vi "day 11 task 1.vi"() -> ()   [LabVIEW 2019]
uses:
  <userlib>/_OpenG.lib/array/array.llb/Search 1D Array (I32)__ogtk.vi
panel:
  out "level of monkey business":i32
  out "Amount of inspections by each monkey":i32[](array[numeric])
  out "Monkeys after 20 rounds":T1(array[cluster])
  out "Monkeys":T2(array[cluster])
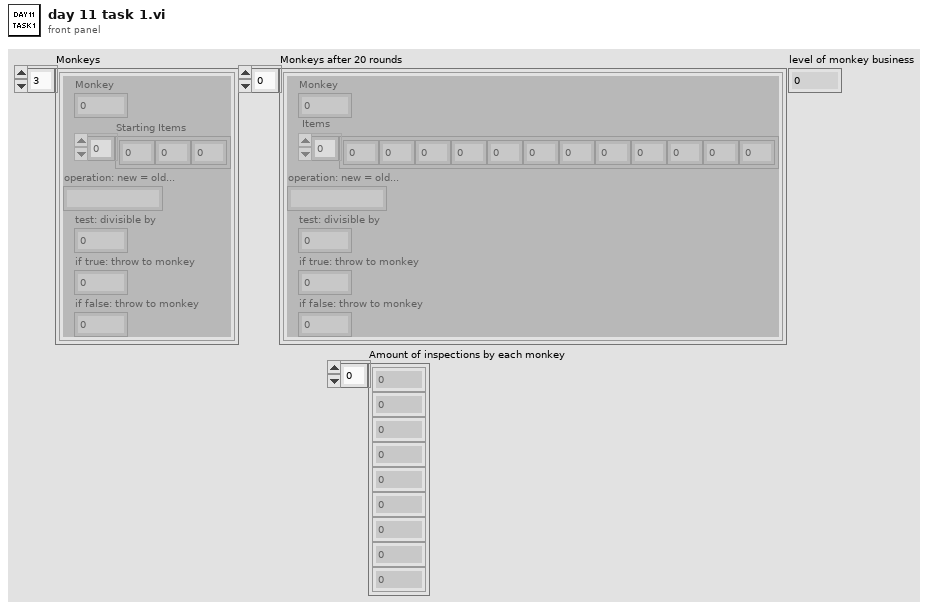
[diagram p1: front panel]
types:
  T1 = cluster{"Monkey":i32, " Items":i32[], "operation: new = old...":string, "test: divisible by":i32, "if true: throw to monkey":i32, "if false: throw to monkey":i32}[]
  T2 = cluster{"Monkey":i32, "Starting Items":i32[], "operation: new = old...":string, "test: divisible by":i32, "if true: throw to monkey":i32, "if false: throw to monkey":i32}[]
  T3 = cluster{"Monkey":i32, "Starting Items":i32[], "operation: new = old...":string, "test: divisible by":i32, "if true: throw to monkey":i32, "if false: throw to monkey":i32}
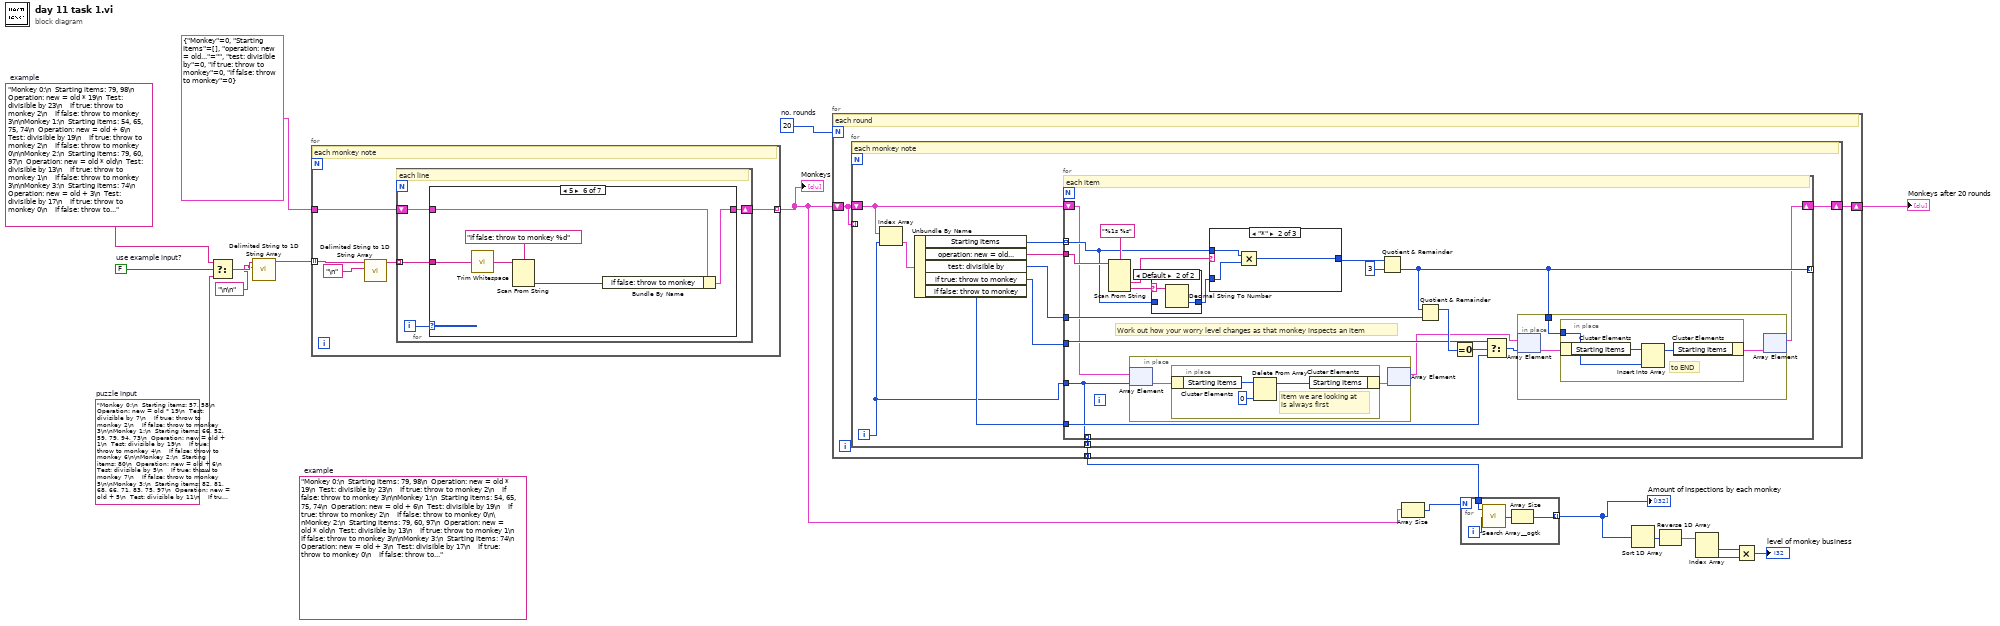
[diagram p0: block diagram]
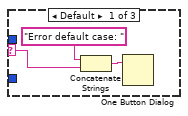
[diagram p3: hidden frame]
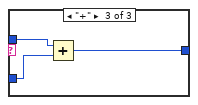
[diagram p4: hidden frame]
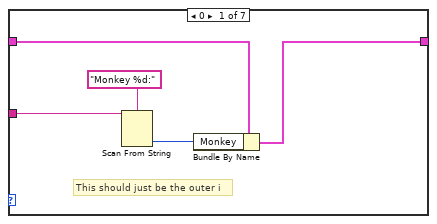
[diagram p5: hidden frame]
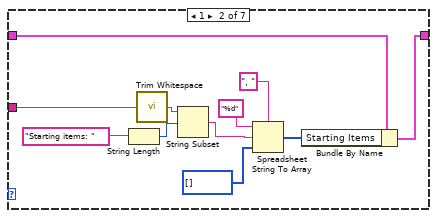
[diagram p6: hidden frame]
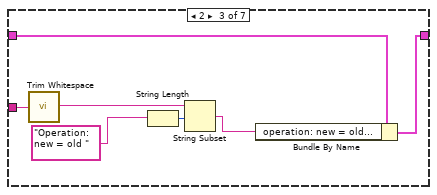
[diagram p7: hidden frame]
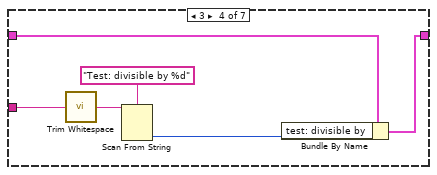
[diagram p8: hidden frame]
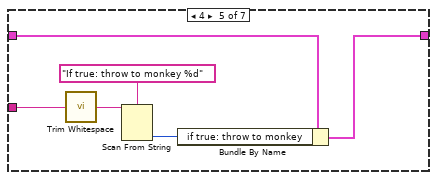
[diagram p9: hidden frame]
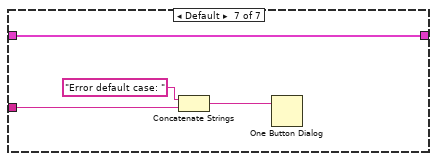
[diagram p10: hidden frame]
diagram:
  w10 = 20  # no. rounds
  (unwired) "Monkey 0:\n  Starting items: 79, 98\n  Operation: new = old * 19\n  Test: divisible by 23\n    If true: throw to monkey 2\n    If false: throw to monkey 3\n\nMonkey 1:\n  Starting items: 54, 65, 75, 74\n  Operation: new = old + 6\n  Test: divisible by 19\n    If true: throw to monkey 2\n    If false: throw to monkey 0\n\nMonkey 2:\n  Starting items: 79, 60, 97\n  Operation: new = old * old\n  Test: divisible by 13\n    If true: throw to monkey 1\n    If false: throw to monkey 3\n\nMonkey 3:\n  Starting items: 74\n  Operation: new = old + 3\n  Test: divisible by 17\n    If true: throw to monkey 0\n    If false: throw to monkey 1"  # example
  w16 = "Monkey 0:\n  Starting items: 79, 98\n  Operation: new = old * 19\n  Test: divisible by 23\n    If true: throw to monkey 2\n    If false: throw to monkey 3\n\nMonkey 1:\n  Starting items: 54, 65, 75, 74\n  Operation: new = old + 6\n  Test: divisible by 19\n    If true: throw to monkey 2\n    If false: throw to monkey 0\n\nMonkey 2:\n  Starting items: 79, 60, 97\n  Operation: new = old * old\n  Test: divisible by 13\n    If true: throw to monkey 1\n    If false: throw to monkey 3\n\nMonkey 3:\n  Starting items: 74\n  Operation: new = old + 3\n  Test: divisible by 17\n    If true: throw to monkey 0\n    If false: throw to monkey 1"  # example
  w17 = FALSE  # use example input?
  w18 = "Monkey 0:\n  Starting items: 57, 58\n  Operation: new = old * 19\n  Test: divisible by 7\n    If true: throw to monkey 2\n    If false: throw to monkey 3\n\nMonkey 1:\n  Starting items: 66, 52, 59, 79, 94, 73\n  Operation: new = old + 1\n  Test: divisible by 19\n    If true: throw to monkey 4\n    If false: throw to monkey 6\n\nMonkey 2:\n  Starting items: 80\n  Operation: new = old + 6\n  Test: divisible by 5\n    If true: throw to monkey 7\n    If false: throw to monkey 5\n\nMonkey 3:\n  Starting items: 82, 81, 68, 66, 71, 83, 75, 97\n  Operation: new = old + 5\n  Test: divisible by 11\n    If true: throw to monkey 5\n    If false: throw to monkey 2\n\nMonkey 4:\n  Starting items: 55, 52, 67, 70, 69, 94, 90\n  Operation: new = old * old\n  Test: divisible by 17\n    If true: throw to monkey 0\n    If false: throw to monkey 3\n\nMonkey 5:\n  Starting items: 69, 85, 89, 91\n  Operation: new = old + 7\n  Test: divisible by 13\n    If true: throw to monkey 1\n    If false: throw to monkey 7\n\nMonkey 6:\n  Starting items: 75, 53, 73, 52, 75\n  Operation: new = old * 7\n  Test: divisible by 2\n    If true: throw to monkey 0\n    If false: throw to monkey 4\n\nMonkey 7:\n  Starting items: 94, 60, 79\n  Operation: new = old + 2\n  Test: divisible by 3\n    If true: throw to monkey 1\n    If false: throw to monkey 6"  # puzzle input
  n1 = Select(t=w16, s=w17, f=w18) -> (s? t:f=w15:string)
  n2 = call <vilib>:"Delimited String to 1D String Array.vi"("delimiter"="\n\n" ("regular expression"), "delimited string"=w15) -> ("string array"=w13:string[])  [unwired: 9 in]
  n3 = for {
    tunnel: w13 -> [w23] mode=indexing
    tunnel: T3 {"Monkey"=0, "Starting Items"=[], "operation: new = old..."="", "test: divisible by"=0, "if true: throw to monkey"=0, "if false: throw to monkey"=0} -> [w22]
    tunnel: [w21] -> w8 mode=indexing
    # "each monkey note"
    n4 = call <vilib>:"Delimited String to 1D String Array.vi"("delimiter"="\n", "delimited string"=w23) -> ("string array"=w20:string[])  [unwired: 9 in]
    n5 = for {
      tunnel: w20 -> [w26] mode=indexing
      shift-right: [w25] -> w21
      shift-left: w22 -> [w24]
      i -> [w27]
      # "each line"
      n6 = case shown="5" w27 {
        tunnel: w26 -> [w32 w40 w50 w54 w60 w66 w70]
        tunnel: [w30 w37 w48 w51 w57 w63 w69] -> w25
        tunnel: w24 -> [w29 w38 w49 w52 w58 w65 w69]
        frame 0 {
          # "This should just be the outer i"
          n7 = Scan From String(format string="Monkey %d:", input string=w32) -> (output 1=w28:i32)  [unwired: 3 in, 3 out]
          n8 = Bundle By Name(cluster=w29, "Monkey"=w28) -> (w30:T3)
        }
        frame 1 {
          n9 = String Length(string="Starting items: " ("format string")) -> (length=w34:i32)
          n10 = call <vilib>:"Trim Whitespace.vi"("string"=w40) -> ("trimmed string"=w33:string)  [unwired: 1 in]
          n11 = String Subset(string=w33, offset (0)=w34) -> (substring=w36:string)  [unwired: 1 in]
          n12 = Spreadsheet String To Array(delimiter (Tab)=", ", format string="%d", spreadsheet string=w36, array type (2D Dbl)=i32[] []) -> (array=w39:i32[])
          n13 = Bundle By Name(cluster=w38, "Starting Items"=w39) -> (w37:T3)
        }
        frame 2 {
          n14 = call <vilib>:"Trim Whitespace.vi"("string"=w50) -> ("trimmed string"=w46:string)  [unwired: 1 in]
          n15 = String Length(string="Operation: new = old " ("format string")) -> (length=w44:i32)
          n16 = String Subset(string=w46, offset (0)=w44) -> (substring=w47:string)  [unwired: 1 in]
          n17 = Bundle By Name(cluster=w49, "operation: new = old..."=w47) -> (w48:T3)
        }
        frame 3 {
          n18 = call <vilib>:"Trim Whitespace.vi"("string"=w54) -> ("trimmed string"=w55:string)  [unwired: 1 in]
          n19 = Scan From String(format string="Test: divisible by %d", input string=w55) -> (output 1=w53:i32)  [unwired: 3 in, 3 out]
          n20 = Bundle By Name(cluster=w52, "test: divisible by"=w53) -> (w51:T3)
        }
        frame 4 {
          n21 = call <vilib>:"Trim Whitespace.vi"("string"=w60) -> ("trimmed string"=w61:string)  [unwired: 1 in]
          n22 = Scan From String(format string="If true: throw to monkey %d", input string=w61) -> (output 1=w59:i32)  [unwired: 3 in, 3 out]
          n23 = Bundle By Name(cluster=w58, "if true: throw to monkey"=w59) -> (w57:T3)
        }
        frame 5 {
          n24 = call <vilib>:"Trim Whitespace.vi"("string"=w66) -> ("trimmed string"=w67:string)  [unwired: 1 in]
          n25 = Scan From String(format string="If false: throw to monkey %d", input string=w67) -> (output 1=w64:i32)  [unwired: 3 in, 3 out]
          n26 = Bundle By Name(cluster=w65, "if false: throw to monkey"=w64) -> (w63:T3)
        }
        frame Default {
          n27 = Concatenate Strings("Error default case: " ("message"), w70) -> (w71:string)
          n28 = One Button Dialog(message=w71) -> ()  [unwired: 1 in, 1 out]
        }
      }
    }
  }
  "Monkeys" <- w8
  n29 = for {
    N: w10 -> [_]
    shift-right: [w75] -> w11
    shift-left: w8 -> [w74]
    tunnel: [w73] -> w7 mode=concatenating
    # "each round"
    n30 = for {
      shift-right: [w81] -> w75
      shift-left: w74 -> [w80]
      tunnel: w74 -> [_] mode=indexing
      tunnel: [w76] -> w73 mode=concatenating
      i -> [w77]
      # "each monkey note"
      n31 = Index Array(array=w80, index=w77) -> (element=w84:T3)
      n32 = Unbundle By Name(w84) -> ("Starting Items"=w85:i32[], "operation: new = old..."=w83:string, "test: divisible by"=w82:i32, "if true: throw to monkey"=w79:i32, "if false: throw to monkey"=w78:i32)
      n33 = for {
        tunnel: w85 -> [w99] mode=indexing
        tunnel: w83 -> [w104]
        tunnel: [w90] -> _ mode=indexing
        tunnel: w82 -> [w96]
        shift-right: [w87] -> w81
        shift-left: w80 -> [w89]
        tunnel: w79 -> [w93]
        tunnel: w78 -> [w92]
        tunnel: w77 -> [w86]
        tunnel: [w86] -> w76 mode=indexing
        # "Work out how your worry level changes as that monkey inspects an item"
        # "each item"
        n34 = Scan From String(format string="%1s %s", input string=w104) -> (output 1=w102:string, output 2=w101:string)  [unwired: 4 in, 3 out]
        n35 = in-place {
          n36 = in-place-array #1(w89, w86) -> (w112:T3)
          n37 = in-place {
            # "item we are looking at \nis always first"
            n38 = in-place-cluster #2(w112) -> ("Starting Items"=w114:i32[])
            n39 = Delete From Array(array=w114, index=0) -> (array with subset deleted=w115:i32[])  [unwired: 1 in, 1 out]
            n40 = in-place-cluster #2("Starting Items"=w115) -> (w111:T3)
          }
          n41 = in-place-array #1(w111) -> (w88:T2)  [unwired: 1 out]
        }
        n42 = case shown="Default" w101 {
          selector: w101 -> [_ w118]
          tunnel: [w116 w117] -> w100
          tunnel: w99 -> [w116 _]
          frame "old" {
          }
          frame Default {
            n43 = Decimal String To Number(string=w118) -> (number=w117:i32)  [unwired: 2 in, 1 out]
          }
        }
        n44 = case shown="\"*\"" w102 {
          selector: w102 -> [w119 _ _]
          tunnel: w100 -> [_ w124 w127]
          tunnel: w99 -> [_ w123 w126]
          tunnel: [_ w122 w125] -> w98
          frame Default {
            n45 = Concatenate Strings("Error default case: " ("message"), w119) -> (w121:string)
            n46 = One Button Dialog(message=w121) -> ()  [unwired: 1 in, 1 out]
          }
          frame "*" {
            n47 = Multiply(x=w123, y=w124) -> (x*y=w122:i32)
          }
          frame "+" {
            n48 = Add(x=w126, y=w127) -> (x+y=w125:i32)
          }
        }
        n49 = Quotient & Remainder(x=w98, y=3) -> (floor(x/y)=w90:i32)  [unwired: 1 out]
        n50 = Quotient & Remainder(x=w90, y=w96) -> (x-y*floor(x/y)=w95:i32)  [unwired: 1 out]
        n51 = Equal To 0?(x=w95) -> (x = 0?=w94:bool)
        n52 = Select(t=w93, s=w94, f=w92) -> (s? t:f=w91:i32)
        n53 = in-place {
          in-place-border: w90 -> [w107]
          n54 = in-place-array #3(w88, w91) -> (w105:T3)
          n55 = in-place {
            in-place-border: w107 -> [w109]
            # "to END"
            n56 = in-place-cluster #4(w105) -> ("Starting Items"=w108:i32[])
            n57 = Insert Into Array(array=w108, new element=w109) -> (w110:i32[])  [unwired: 1 in]
            n58 = in-place-cluster #4("Starting Items"=w110) -> (w106:T3)
          }
          n59 = in-place-array #3(w106) -> (w87:T2)  [unwired: 1 out]
        }
      }
    }
  }
  "Monkeys after 20 rounds" <- w11
  n60 = Array Size(array=w8) -> (size(s)=w9:i32)
  n61 = for {
    N: w9 -> [_]
    tunnel: w7 -> [w131]
    tunnel: [w128] -> w6 mode=indexing
    i -> [w130]
    n62 = call-poly <userlib>:"Search Array__ogtk.vi"("Array"=w131, "Element Data"=w130) -> ("Indices of Elements"=w129:i32[])  [unwired: 7 in]
    n63 = Array Size(array=w129) -> (size(s)=w128:i32)
  }
  "Amount of inspections by each monkey" <- w6
  n64 = Sort 1D Array(array=w6) -> (sorted array=w2:i32[])
  n65 = Reverse 1D Array(array=w2) -> (reversed array=w1:i32[])
  n66 = Index Array(array=w1) -> (element #1=w5:i32, element #2=w4:i32)  [unwired: 2 in]
  n67 = Multiply(x=w5, y=w4) -> (x*y=→"level of monkey business":i32)
